vi "repPrepareFreeBallPlayVSS.vi"(8 "error in (no error)":errorcluster, 9 "Game in 2":refnum<class "Game.lvclass">, 10 "RobotPlacement":T1(array[cluster]), 11 "PrepareFreeBallPlayVSS in":refnum<class "PrepareFreeBallPlayVSS.lvclass">) -> (0 "error out":errorcluster, 2 "RobotPlacement 2":T1(array[cluster]), 3 "PrepareFreeBallPlayVSS out":refnum<class "PrepareFreeBallPlayVSS.lvclass">)   [LabVIEW 2023, in "PrepareFreeBallPlayVSS.lvclass"]
uses:
  PrepareFreeBallPlayVSS.lvclass
  Game_class/Game.lvclass
  Game_class/Game.lvclass/Game.ctl
  Object_class/Object.lvclass/Object.ctl
  Team_class/Team.lvclass/Team.ctl
  Robot_class/Robot.lvclass/Robot.ctl
  Utilities_class/Utilities.lvclass
  Object_class/Read x.vi
  Object_class/Read y.vi
  Robot_class/Read orientation.vi
  Game_class/Read FieldRef.vi
  Game_class/Read BallRef.vi
  Game_class/Read KeeperTeam.vi
  Team_class/Read RobotRef.vi
  Ally_class/Ally.lvclass
  Ball_class/Ball.lvclass
  Robot_class/Robot.lvclass
  Field_class/Field.lvclass
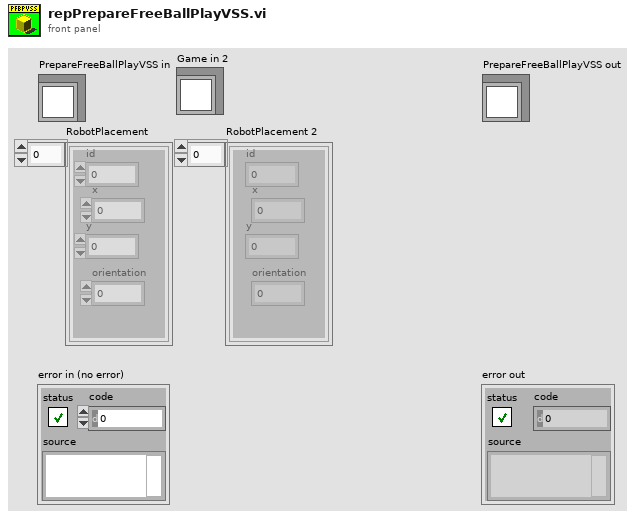
[diagram p1: front panel]
types:
  T1 = cluster{"id":i32, "x":dbl, "y":dbl, "orientation":dbl}[]
  T2 = cluster{"id":i32, "x":dbl, "y":dbl, "orientation":dbl}
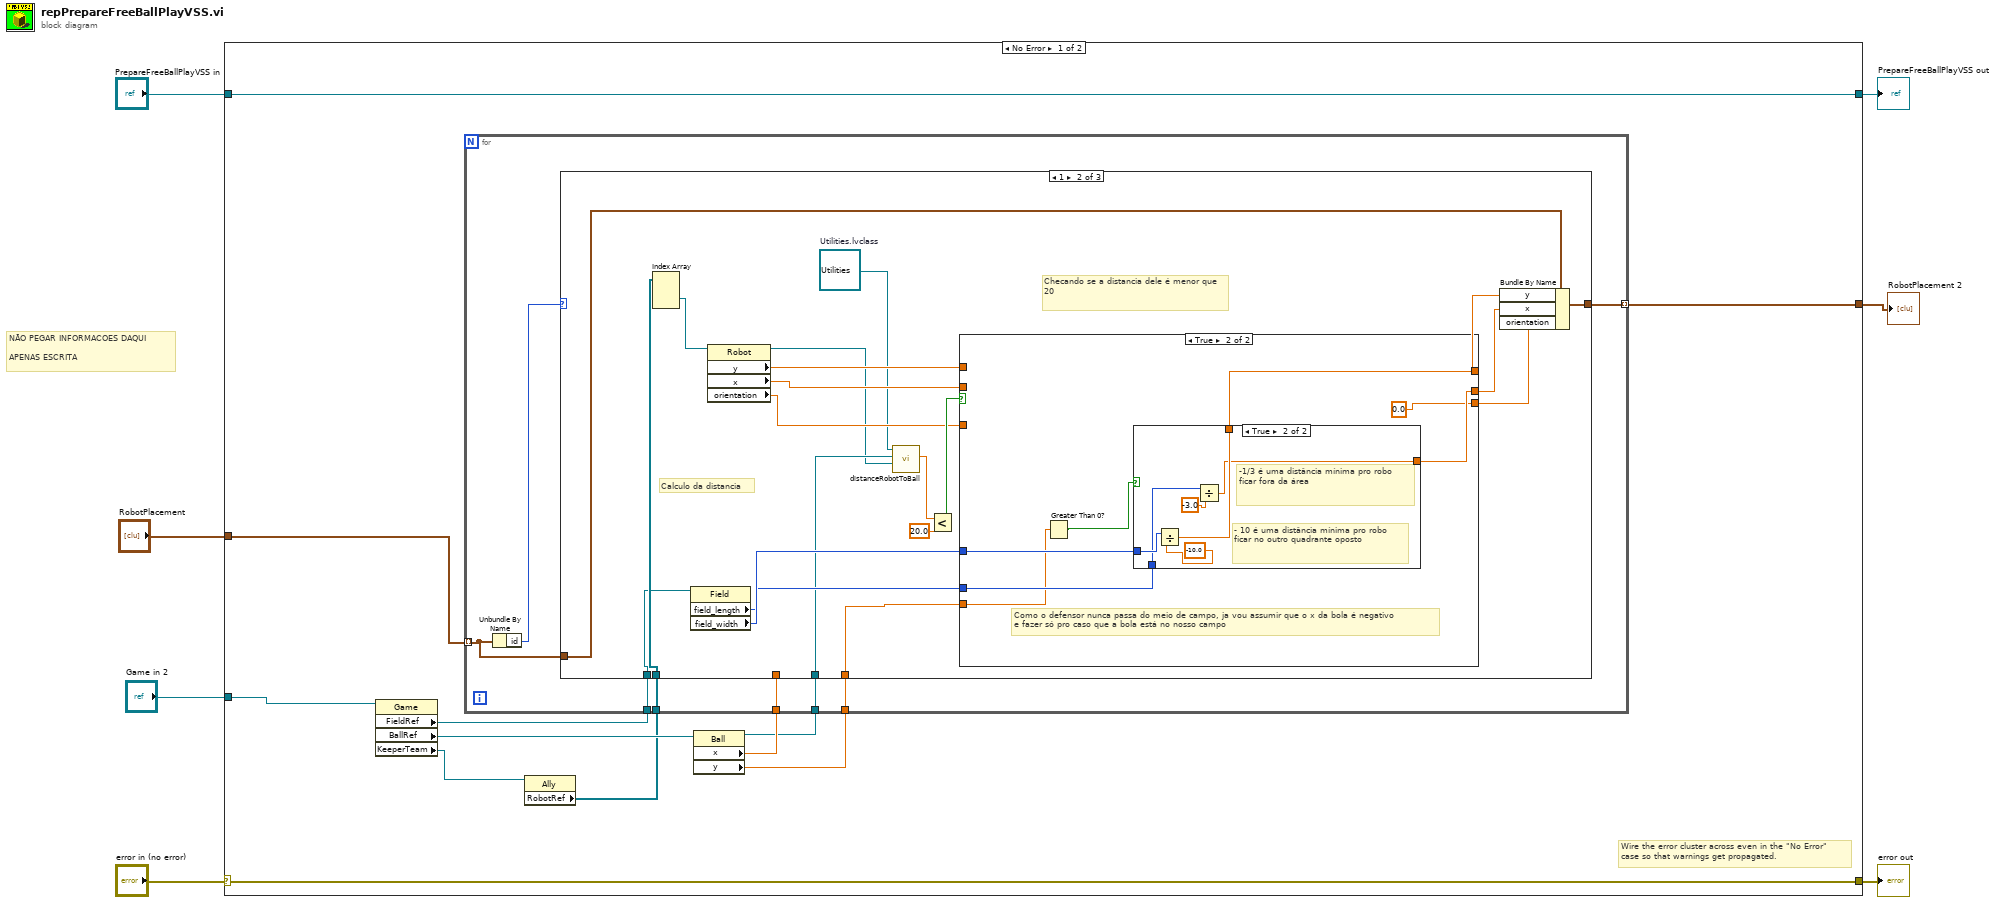
[diagram p0: block diagram]
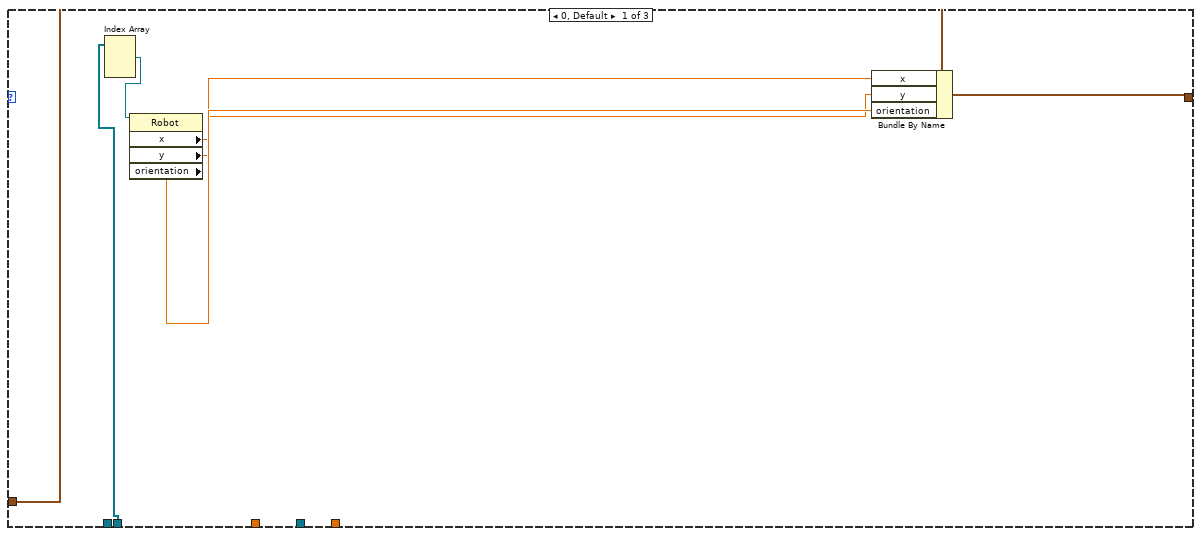
[diagram p2: hidden frame]
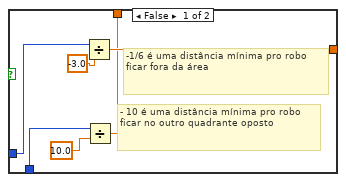
[diagram p4: hidden frame]
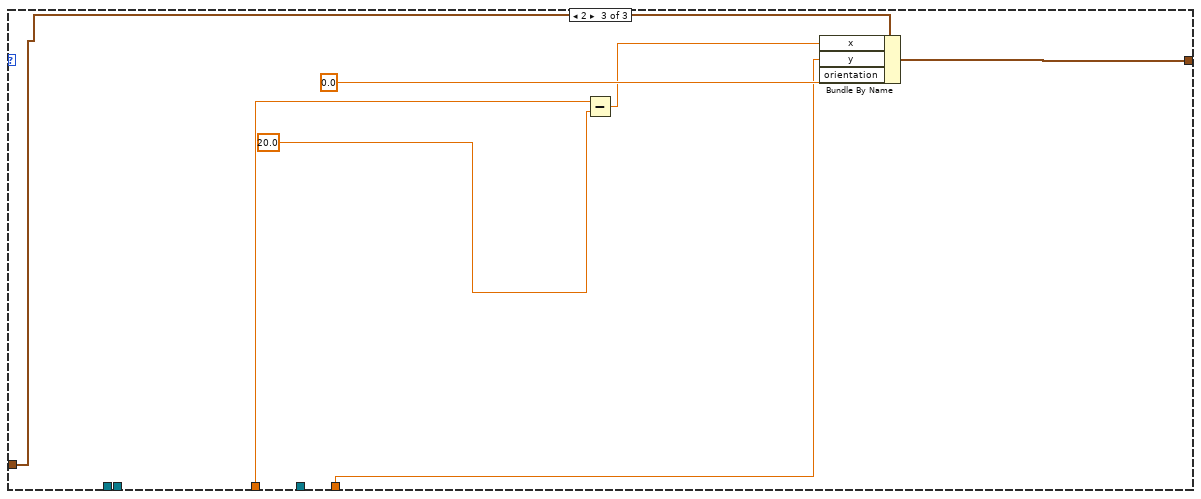
[diagram p5: hidden frame]
diagram:
  # "NÃO PEGAR INFORMACOES DAQUI\n\nAPENAS ESCRITA"
  n1 = case shown="No Error" "error in (no error)" {
    selector: "error in (no error)" -> [w18 w85]
    tunnel: [w18 w85] -> w6
    tunnel: [w19 w84] -> w4
    tunnel: "PrepareFreeBallPlayVSS in" -> [w19 w84]
    tunnel: "RobotPlacement" -> [w16 _]
    tunnel: "Game in 2" -> [w17 _]
    tunnel: [w15 _] -> w1
    frame No Error {
      # "Wire the error cluster across even in the \"No Error\"\ncase so that warnings get propagated."
      n2 = property class="Game"(reference=w17) -> ("FieldRef"=w14:refnum<class "Field.lvclass">, "BallRef"=w13:refnum<class "Ball.lvclass">, "KeeperTeam"=w12:refnum<class "Ally.lvclass">)  [unwired: 1 in, 2 out]
      n3 = property class="Ally"(reference=w12) -> ("RobotRef"=w11:refnum<class "Robot.lvclass">[])  [unwired: 1 in, 2 out]
      n4 = property class="Ball"(reference=w13) -> (reference out=w8:refnum<class "Ball.lvclass">, "x"=w10:dbl, "y"=w9:dbl)  [unwired: 1 in, 1 out]
      n5 = for {
        tunnel: w16 -> [w26] mode=indexing
        tunnel: [w25] -> w15 mode=indexing
        tunnel: w14 -> [w24]
        tunnel: w11 -> [w23]
        tunnel: w10 -> [w22]
        tunnel: w9 -> [w21]
        tunnel: w8 -> [w20]
        n6 = Unbundle By Name(w26) -> ("id"=w27:i32)
        n7 = case shown="1" w27 {
          tunnel: w26 -> [w34 w54 w83]
          tunnel: [w33 w53 w82] -> w25
          tunnel: w24 -> [_ w45 _]
          tunnel: w23 -> [w29 w52 _]
          tunnel: w22 -> [_ _ w78]
          tunnel: w21 -> [_ w39 w77]
          tunnel: w20 -> [_ w37 _]
          frame 0, Default {
            n8 = Index Array(array=w29) -> (element #1=w28:refnum<class "Robot.lvclass">)  [unwired: 3 in, 2 out]
            n9 = property class="Robot"(reference=w28) -> ("x"=w30:dbl, "y"=w31:dbl, "orientation"=w32:dbl)  [unwired: 1 in, 2 out]
            n10 = Bundle By Name(cluster=w34, "x"=w30, "y"=w31, "orientation"=w32) -> (w33:T2)
          }
          frame 1 {
            w38 = refnum<class "Utilities.lvclass"> refnum  # Utilities.lvclass
            # "Calculo da distancia"
            # "Checando se a distancia dele é menor que 20"
            n11 = Index Array(array=w52) -> (element #2=w51:refnum<class "Robot.lvclass">)  [unwired: 3 in, 2 out]
            n12 = property class="Field"(reference=w45) -> ("field_length"=w43:i32, "field_width"=w44:i32)  [unwired: 1 in, 2 out]
            n13 = property class="Robot"(reference=w51) -> (reference out=w36:refnum<class "Robot.lvclass">, "y"=w40:dbl, "x"=w41:dbl, "orientation"=w47:dbl)  [unwired: 1 in, 1 out]
            n14 = call "distanceRobotToBall.vi"("Robot"=w36, "Ball"=w37, "Utilities in"=w38) -> ("Distance Robot To Ball"=w35:dbl)  [unwired: 6 in, 2 out]
            n15 = Less?(x=w35, y=20.0) -> (x < y?=w50:bool)
            n16 = case shown="True" w50 {
              tunnel: [w57 w63] -> w49
              tunnel: w40 -> [w57 _]
              tunnel: [w56 w60] -> w48
              tunnel: w41 -> [w56 _]
              tunnel: [w55 0.0] -> w46
              tunnel: w47 -> [w55 _]
              tunnel: w44 -> [_ w62]
              tunnel: w43 -> [_ w61]
              tunnel: w39 -> [_ w58]
              frame False {
              }
              frame True {
                # "Como o defensor nunca passa do meio de campo, ja vou assumir que o x da bola é negativo\ne fazer só pro caso que a bola está no nosso campo"
                n17 = Greater Than 0?(x=w58) -> (x > 0?=w64:bool)
                n18 = case shown="True" w64 {
                  tunnel: [w66 w75] -> w63
                  tunnel: w62 -> [w65 w74]
                  tunnel: w61 -> [w68 w71]
                  tunnel: [w67 w72] -> w60
                  frame False {
                    # "- 10 é uma distância mínima pro robo\nficar no outro quadrante oposto"
                    # "-1/6 é uma distância mínima pro robo\nficar fora da área"
                    n19 = Divide(x=w65, y=-3.0) -> (x/y=w67:dbl)
                    n20 = Divide(x=w68, y=10.0) -> (x/y=w66:dbl)
                  }
                  frame True {
                    # "-1/3 é uma distância mínima pro robo\nficar fora da área"
                    # "- 10 é uma distância mínima pro robo\nficar no outro quadrante oposto"
                    n21 = Divide(x=w74, y=-10.0) -> (x/y=w75:dbl)
                    n22 = Divide(x=w71, y=-3.0) -> (x/y=w72:dbl)
                  }
                }
              }
            }
            n23 = Bundle By Name(cluster=w54, "y"=w49, "x"=w48, "orientation"=w46) -> (w53:T2)
          }
          frame 2 {
            n24 = Subtract(x=w78, y=20.0 ("x")) -> (x-y=w79:dbl)
            n25 = Bundle By Name(cluster=w83, "x"=w79, "y"=w77, "orientation"=0.0) -> (w82:T2)
          }
        }
      }
    }
    frame Error {
    }
  }
  "error out" <- w6
  "PrepareFreeBallPlayVSS out" <- w4
  "RobotPlacement 2" <- w1
